vi "change vi properties.vi"() -> ()   [LabVIEW 2019]
panel:
  out "Numeric":i32
  out "Number of Files":i32
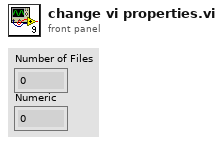
[diagram p1: front panel]
types:
  T1 = enum16{"Share clones between instances", "Preallocate clone for each instance"}
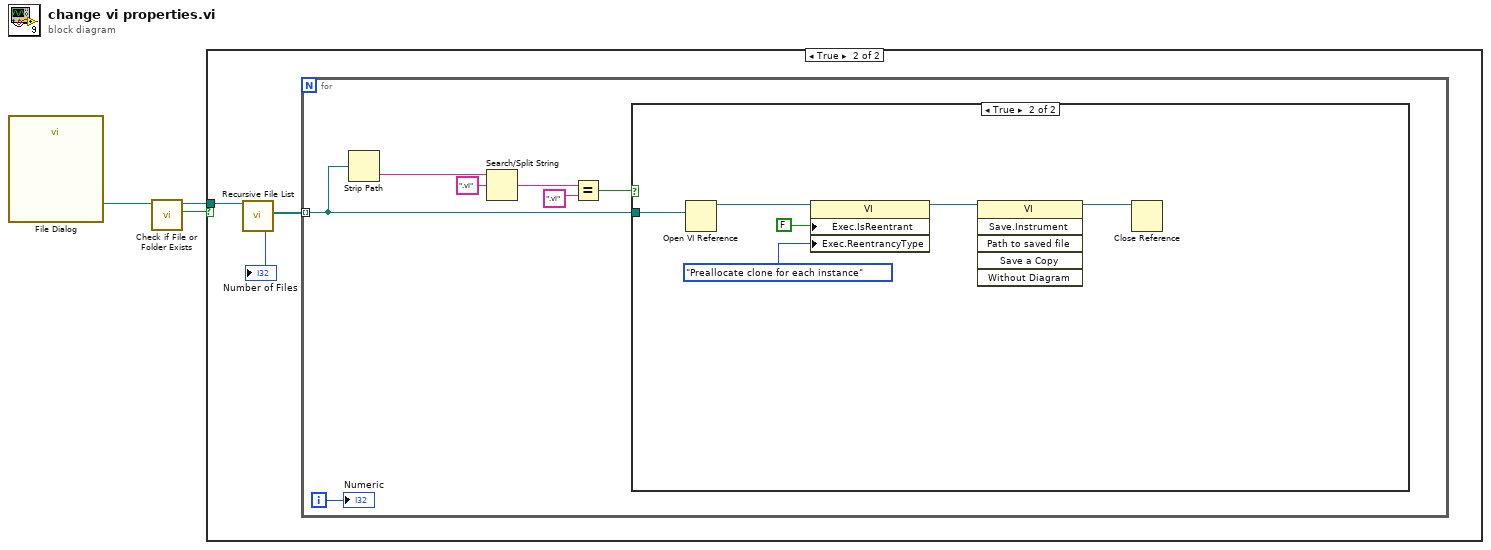
[diagram p0: block diagram]
diagram:
  n1 = call "File Dialog"() -> ("selected path"=w3:path)  [unwired: 12 in, 3 out]
  n2 = call <vilib>:"Check if File or Folder Exists.vi"("path"=w3) -> ("file or folder exists?"=w2:bool, "dup path"=w1:path)  [unwired: 8 in, 1 out]
  n3 = case shown="True" w2 {
    tunnel: w1 -> [_ w6]
    frame False {
    }
    frame True {
      n4 = call <vilib>:"Recursive File List.vi"("Folder Path"=w6) -> ("Number of Files"=→"Number of Files":i32, "All Files in Dir"=w5:path[])  [unwired: 6 in, 3 out]
      n5 = for {
        tunnel: w5 -> [w8] mode=indexing
        i -> [w7]
        n6 = Strip Path(path=w8) -> (name=w13:string)  [unwired: 1 out]
        n7 = Search/Split String(string=w13, search string/char (-)=".vi") -> (match + rest of string=w11:string)  [unwired: 1 in, 2 out]
        n8 = Equal?(x=w11, y=".vi" ("search string/char (-)")) -> (x = y?=w9:bool)
        n9 = case shown="True" w9 {
          tunnel: w8 -> [_ w19]
          frame False {
          }
          frame True {
            n10 = Open VI Reference(vi path=w19) -> (vi reference=w18:refnum<vi>)  [unwired: 5 in, 1 out]
            n11 = property class="VI"(reference=w18, "Exec.IsReentrant"=FALSE ("Execution:Is Reentrant"), "Exec.ReentrancyType"=T1."Preallocate clone for each instance" ("Execution:Reentrancy Type")) -> (reference out=w15:refnum<vi>)  [unwired: 1 in, 1 out]
            n12 = invoke class="VI" method="Save.Instrument"(reference=w15) -> (reference out=w14:refnum<vi>)  [unwired: 5 in, 5 out]
            n13 = Close Reference(reference=w14) -> ()  [unwired: 1 in, 1 out]
          }
        }
        "Numeric" <- w7
      }
    }
  }
